vi "IECMemory.AlphaConv.vi"(7 "String":string) -> (8 "Numeric":i32)   [LabVIEW 2014, in "IECMemory.lvlib"]
doc: "This vi can be used to convert letters to numbers.\na=A=0..z=Z=25."
uses:
  IECMemory.lvlib
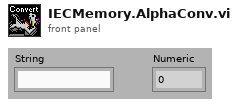
[diagram p1: front panel]
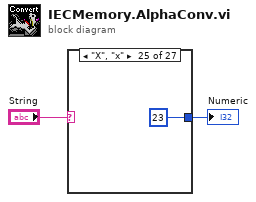
[diagram p0: block diagram]
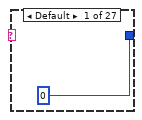
[diagram p2: hidden frame]
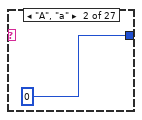
[diagram p3: hidden frame]
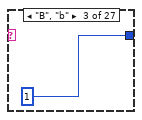
[diagram p4: hidden frame]
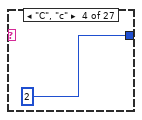
[diagram p5: hidden frame]
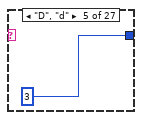
[diagram p6: hidden frame]
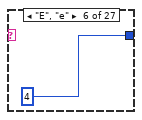
[diagram p7: hidden frame]
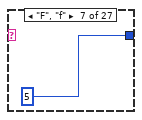
[diagram p8: hidden frame]
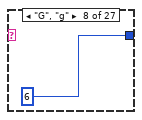
[diagram p9: hidden frame]
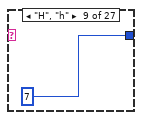
[diagram p10: hidden frame]
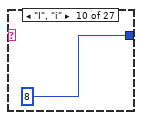
[diagram p11: hidden frame]
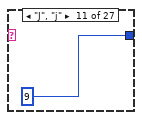
[diagram p12: hidden frame]
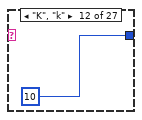
[diagram p13: hidden frame]
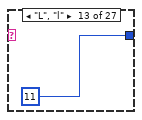
[diagram p14: hidden frame]
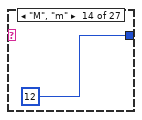
[diagram p15: hidden frame]
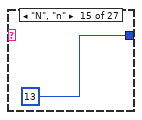
[diagram p16: hidden frame]
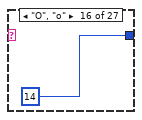
[diagram p17: hidden frame]
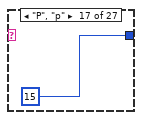
[diagram p18: hidden frame]
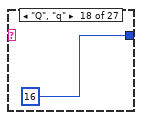
[diagram p19: hidden frame]
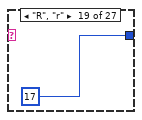
[diagram p20: hidden frame]
diagram:
  n1 = case shown="\"X\", \"x\"" "String" {
    tunnel: [0 0 1 2 3 4 5 6 7 8 9 10 11 12 13 14 15 16 17 18 19 20 21 22 23 25 25] -> w1
    frame Default {
    }
    frame "A", "a" {
    }
    frame "B", "b" {
    }
    frame "C", "c" {
    }
    frame "D", "d" {
    }
    frame "E", "e" {
    }
    frame "F", "f" {
    }
    frame "G", "g" {
    }
    frame "H", "h" {
    }
    frame "I", "i" {
    }
    frame "J", "j" {
    }
    frame "K", "k" {
    }
    frame "L", "l" {
    }
    frame "M", "m" {
    }
    frame "N", "n" {
    }
    frame "O", "o" {
    }
    frame "P", "p" {
    }
    frame "Q", "q" {
    }
    frame "R", "r" {
    }
    frame "S", "s" {
    }
    frame "T", "t" {
    }
    frame "U", "u" {
    }
    frame "V", "v" {
    }
    frame "W", "w" {
    }
    frame "X", "x" {
    }
    frame "Y", "y" {
    }
    frame "Z", "z" {
    }
  }
  "Numeric" <- w1
